vi "figure 8 or loop.vi"() -> ()   [LabVIEW 2014]
doc: "\"Discrete LED demo.vi\" -- Demonstrate a discrete LED connected to a digital output.\n\nInstructions:\n\n-- Click the 'enable blinker' button to toggle between blinking mode\nand static mode.\n-- In static mode, click the 'digital level' button to set the state of the\ndigital output.\n-- The 'digital output state' LED indicator shows the state of the\ndigital output (on = high, off = low)."
uses:
  <vilib>/myRIO/Common/Instrument Driver Framework/myRIO v1.0/UART/vis/myRIO v1.0 Close UART.vi
  <vilib>/Utility/error.llb/Error Cluster From Error Code.vi
  <vilib>/myRIO/Common/Instrument Driver Framework/myRIO v1.0/DIO/vis/myRIO v1.0 Write DIO.vi
  <vilib>/myRIO/Common/Instrument Driver Framework/Utilities/vis/FPGA Ref Manager.vi
  <vilib>/myRIO/Common/Instrument Driver Framework/myRIO v1.0/myRIO v1.0 Reset FPGA.vi
  <vilib>/myRIO/Common/Instrument Driver Framework/myRIO v1.0/IRQ/vis/myRIO v1.0 IRQ Info FGV.vi
  <vilib>/myRIO/Common/Instrument Driver Framework/myRIO v1.0/IRQ/vis/myRIO v1.0 Timer IRQ Info FGV.vi
  <vilib>/myRIO/Common/Instrument Driver Framework/myRIO v1.0/IRQ/vis/myRIO v1.0 ISR Agent.vi
  <vilib>/myRIO/Instrument Drivers/Utilities/Utilities.lvlib
  <vilib>/myRIO/Instrument Drivers/Onboard IO/DIO/DIO.lvlib
panel:
  in  "Numeric":dbl
  in  "reverse":bool
  in  "figure 8":bool
  in  "error in (no error)":errorcluster
  in  "[ESC]":bool
  # "7-Segment LED demo"
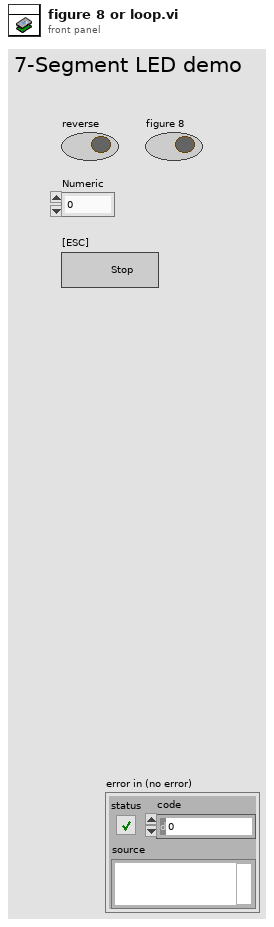
[diagram p1: front panel]
types:
  T1 = typedef "DIO.lvlib/DIO Reference.ctl" = cluster{"myRIO Reference":T2, "DIO Channels List":T6}
  T2 = typedef "myRIO Generic Hardware Reference.ctl" = cluster{"myRIO Model":T3, "myRIO Hardware Reference":T4}
  T3 = typedef "Hardware Version Enum.ctl" = enum16{"Unknown", "myRIO-1900", "myRIO-1950"}
  T4 = typedef "myRIO v1.0 Reference.ctl" = cluster{"Generic FPGA Reference":T5, "Allow multiple opens":bool}
  T5 = typedef "Generic FPGA Reference.ctl" = refnum<k20>
  T6 = typedef "DIO Channels List.ctl" = T7[]
  T7 = typedef "DIO Channels Enum.ctl" = enum16{"Not Connected", "C/DIO0", "C/DIO1", "C/DIO2", "C/DIO3", "C/DIO4", "C/DIO5", "C/DIO6", "C/DIO7", "A/DIO0", "A/DIO1", "A/DIO2", "A/DIO3", "A/DIO4", "A/DIO5", "A/DIO6", "A/DIO7", "A/DIO8", "A/DIO9", "A/DIO10", "A/DIO11", "A/DIO12", "A/DIO13", "A/DIO14", "A/DIO15", "B/DIO0", "B/DIO1", "B/DIO2", "B/DIO3", "B/DIO4", "B/DIO5", "B/DIO6", "B/DIO7", "B/DIO8", "B/DIO9", "B/DIO10", "B/DIO11", "B/DIO12", "B/DIO13", "B/DIO14", "B/DIO15", "LED0", "LED1", "LED2", "LED3", "Button0"}
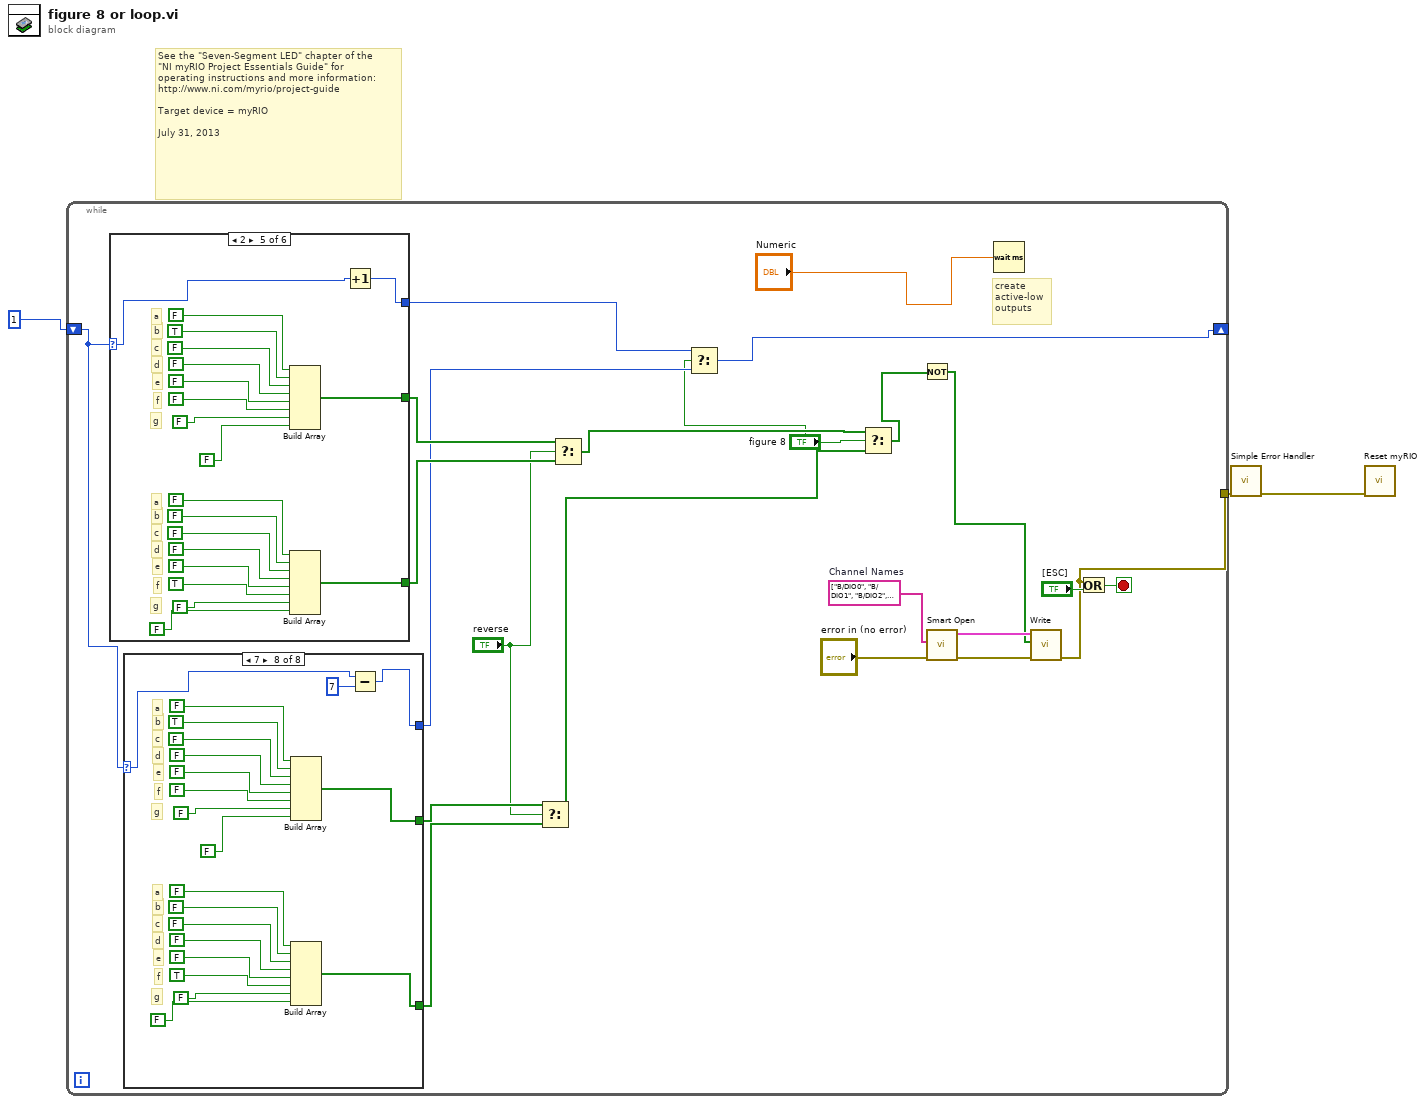
[diagram p0: block diagram]
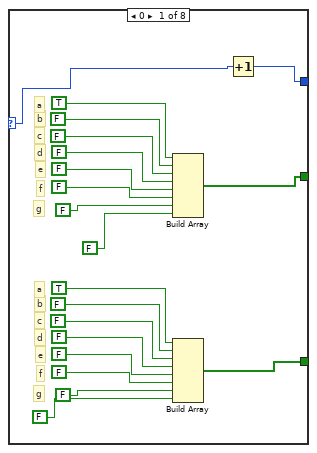
[diagram p2: hidden frame]
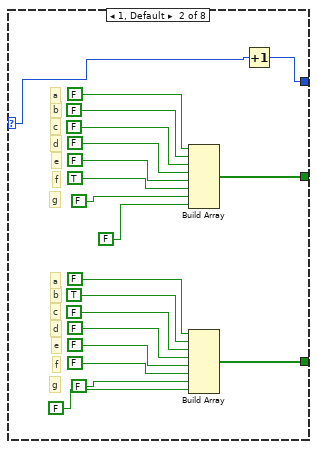
[diagram p3: hidden frame]
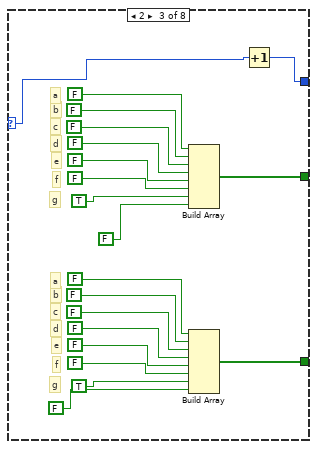
[diagram p4: hidden frame]
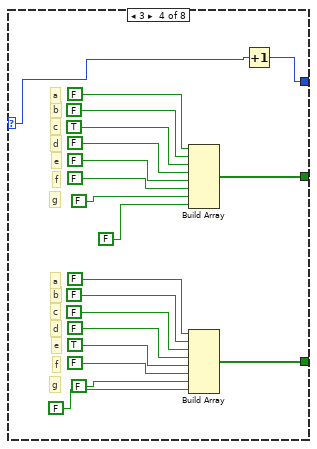
[diagram p5: hidden frame]
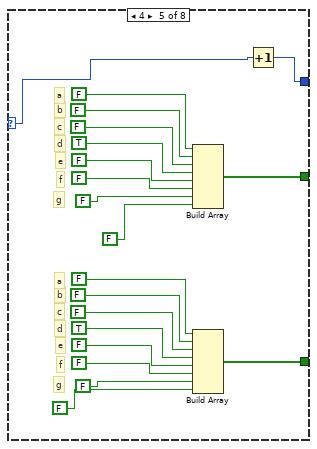
[diagram p6: hidden frame]
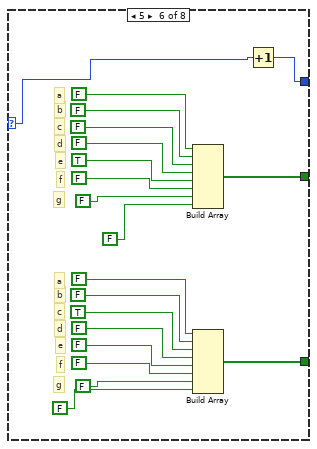
[diagram p7: hidden frame]
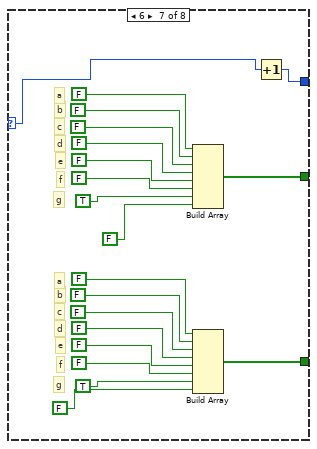
[diagram p8: hidden frame]
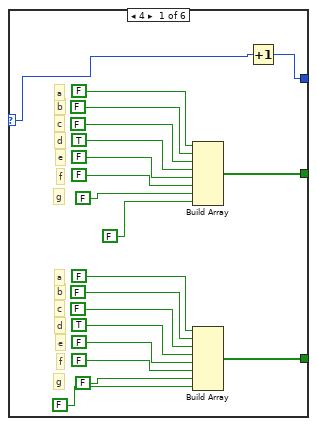
[diagram p9: hidden frame]
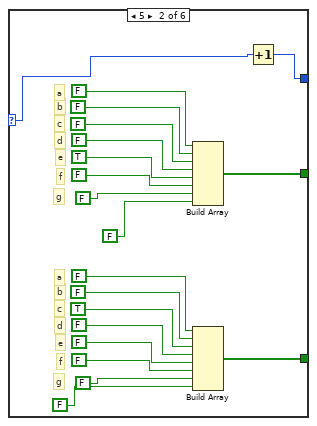
[diagram p10: hidden frame]
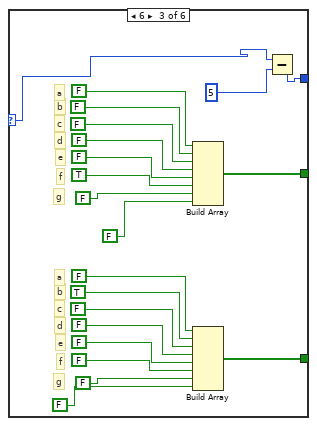
[diagram p11: hidden frame]
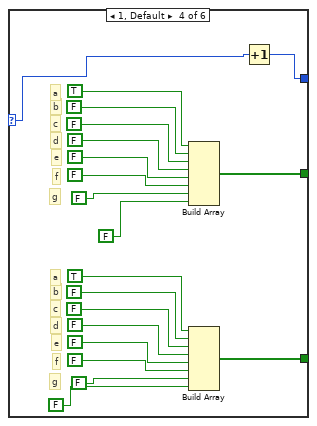
[diagram p12: hidden frame]
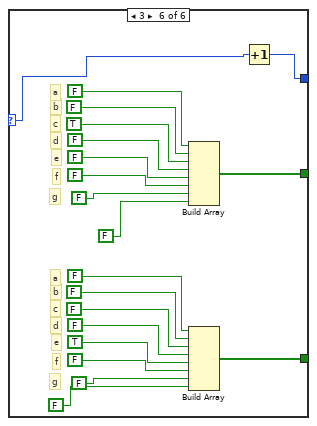
[diagram p13: hidden frame]
diagram:
  # "See the \"Seven-Segment LED\" chapter of the\n\"NI myRIO Project Essentials Guide\" for\noperating instructions and more information: \nhttp://www.ni.com/myrio/project-guide\n\nTarget device = myRIO\n\nJuly 31, 2013"
  n1 = while {
    tunnel: [w19] -> w3
    shift-right: [w7] -> _
    shift-left: 1 -> [w16]
    stop <- w25 stop-if-true
    w23 = tag[] ["B/DIO0", "B/DIO1", "B/DIO2", "B/DIO3", "B/DIO4", "B/DIO5", "B/DIO6", "B/DIO7"]  # Channel Names
    # "create\nactive-low\noutputs"
    n2 = case shown="2" w16 {
      selector: w16 -> [w189 w209 w229 w248 w268 w288]
      tunnel: [w198 w218 w228 w249 w269 w289] -> w8
      tunnel: [w188 w208 w231 w251 w271 w291] -> w11
      tunnel: [w187 w207 w230 w250 w270 w290] -> w10
      frame 4 {
        # "g"
        # "f"
        # "e"
        # "d"
        # "c"
        # "b"
        # "a"
        # "g"
        # "f"
        # "e"
        # "d"
        # "c"
        # "b"
        # "a"
        n3 = Build Array(FALSE, FALSE, FALSE, TRUE, FALSE, FALSE, FALSE, FALSE) -> (w187:bool[])
        n4 = Build Array(FALSE, FALSE, FALSE, TRUE, FALSE, FALSE, FALSE, FALSE) -> (w188:bool[])
        n5 = Increment(x=w189) -> (x+1=w198:i32)
      }
      frame 5 {
        # "g"
        # "f"
        # "e"
        # "d"
        # "c"
        # "b"
        # "a"
        # "g"
        # "f"
        # "e"
        # "d"
        # "c"
        # "b"
        # "a"
        n6 = Build Array(FALSE, FALSE, FALSE, FALSE, TRUE, FALSE, FALSE, FALSE) -> (w207:bool[])
        n7 = Build Array(FALSE, FALSE, TRUE, FALSE, FALSE, FALSE, FALSE, FALSE) -> (w208:bool[])
        n8 = Increment(x=w209) -> (x+1=w218:i32)
      }
      frame 6 {
        # "g"
        # "f"
        # "e"
        # "d"
        # "c"
        # "b"
        # "a"
        # "g"
        # "f"
        # "e"
        # "d"
        # "c"
        # "b"
        # "a"
        n9 = Build Array(FALSE, FALSE, FALSE, FALSE, FALSE, TRUE, FALSE, FALSE) -> (w230:bool[])
        n10 = Build Array(FALSE, TRUE, FALSE, FALSE, FALSE, FALSE, FALSE, FALSE) -> (w231:bool[])
        n11 = Subtract(x=w229, y=5) -> (x-y=w228:i32)
      }
      frame 1, Default {
        # "g"
        # "f"
        # "e"
        # "d"
        # "c"
        # "b"
        # "a"
        # "g"
        # "f"
        # "e"
        # "d"
        # "c"
        # "b"
        # "a"
        n12 = Build Array(TRUE, FALSE, FALSE, FALSE, FALSE, FALSE, FALSE, FALSE) -> (w250:bool[])
        n13 = Build Array(TRUE, FALSE, FALSE, FALSE, FALSE, FALSE, FALSE, FALSE) -> (w251:bool[])
        n14 = Increment(x=w248) -> (x+1=w249:i32)
      }
      frame 2 {
        # "g"
        # "f"
        # "e"
        # "d"
        # "c"
        # "b"
        # "a"
        # "g"
        # "f"
        # "e"
        # "d"
        # "c"
        # "b"
        # "a"
        n15 = Build Array(FALSE, TRUE, FALSE, FALSE, FALSE, FALSE, FALSE, FALSE) -> (w270:bool[])
        n16 = Build Array(FALSE, FALSE, FALSE, FALSE, FALSE, TRUE, FALSE, FALSE) -> (w271:bool[])
        n17 = Increment(x=w268) -> (x+1=w269:i32)
      }
      frame 3 {
        # "g"
        # "f"
        # "e"
        # "d"
        # "c"
        # "b"
        # "a"
        # "g"
        # "f"
        # "e"
        # "d"
        # "c"
        # "b"
        # "a"
        n18 = Build Array(FALSE, FALSE, TRUE, FALSE, FALSE, FALSE, FALSE, FALSE) -> (w290:bool[])
        n19 = Build Array(FALSE, FALSE, FALSE, FALSE, TRUE, FALSE, FALSE, FALSE) -> (w291:bool[])
        n20 = Increment(x=w288) -> (x+1=w289:i32)
      }
    }
    n21 = case shown="7" w16 {
      selector: w16 -> [w26 w46 w66 w86 w108 w128 w147 w168]
      tunnel: [w27 w47 w67 w87 w117 w137 w146 w167] -> w9
      tunnel: [w28 w49 w69 w89 w107 w127 w149 w169] -> w15
      tunnel: [w29 w48 w68 w88 w106 w126 w148 w170] -> w14
      frame 0 {
        # "g"
        # "f"
        # "e"
        # "d"
        # "c"
        # "b"
        # "a"
        # "g"
        # "f"
        # "e"
        # "d"
        # "c"
        # "b"
        # "a"
        n22 = Build Array(TRUE, FALSE, FALSE, FALSE, FALSE, FALSE, FALSE, FALSE) -> (w29:bool[])
        n23 = Build Array(TRUE, FALSE, FALSE, FALSE, FALSE, FALSE, FALSE, FALSE) -> (w28:bool[])
        n24 = Increment(x=w26) -> (x+1=w27:i32)
      }
      frame 1, Default {
        # "g"
        # "f"
        # "e"
        # "d"
        # "c"
        # "b"
        # "a"
        # "g"
        # "f"
        # "e"
        # "d"
        # "c"
        # "b"
        # "a"
        n25 = Build Array(FALSE, FALSE, FALSE, FALSE, FALSE, TRUE, FALSE, FALSE) -> (w48:bool[])
        n26 = Build Array(FALSE, TRUE, FALSE, FALSE, FALSE, FALSE, FALSE, FALSE) -> (w49:bool[])
        n27 = Increment(x=w46) -> (x+1=w47:i32)
      }
      frame 2 {
        # "g"
        # "f"
        # "e"
        # "d"
        # "c"
        # "b"
        # "a"
        # "g"
        # "f"
        # "e"
        # "d"
        # "c"
        # "b"
        # "a"
        n28 = Build Array(FALSE, FALSE, FALSE, FALSE, FALSE, FALSE, TRUE, FALSE) -> (w68:bool[])
        n29 = Build Array(FALSE, FALSE, FALSE, FALSE, FALSE, FALSE, TRUE, FALSE) -> (w69:bool[])
        n30 = Increment(x=w66) -> (x+1=w67:i32)
      }
      frame 3 {
        # "g"
        # "f"
        # "e"
        # "d"
        # "c"
        # "b"
        # "a"
        # "g"
        # "f"
        # "e"
        # "d"
        # "c"
        # "b"
        # "a"
        n31 = Build Array(FALSE, FALSE, TRUE, FALSE, FALSE, FALSE, FALSE, FALSE) -> (w88:bool[])
        n32 = Build Array(FALSE, FALSE, FALSE, FALSE, TRUE, FALSE, FALSE, FALSE) -> (w89:bool[])
        n33 = Increment(x=w86) -> (x+1=w87:i32)
      }
      frame 4 {
        # "g"
        # "f"
        # "e"
        # "d"
        # "c"
        # "b"
        # "a"
        # "g"
        # "f"
        # "e"
        # "d"
        # "c"
        # "b"
        # "a"
        n34 = Build Array(FALSE, FALSE, FALSE, TRUE, FALSE, FALSE, FALSE, FALSE) -> (w106:bool[])
        n35 = Build Array(FALSE, FALSE, FALSE, TRUE, FALSE, FALSE, FALSE, FALSE) -> (w107:bool[])
        n36 = Increment(x=w108) -> (x+1=w117:i32)
      }
      frame 5 {
        # "g"
        # "f"
        # "e"
        # "d"
        # "c"
        # "b"
        # "a"
        # "g"
        # "f"
        # "e"
        # "d"
        # "c"
        # "b"
        # "a"
        n37 = Build Array(FALSE, FALSE, FALSE, FALSE, TRUE, FALSE, FALSE, FALSE) -> (w126:bool[])
        n38 = Build Array(FALSE, FALSE, TRUE, FALSE, FALSE, FALSE, FALSE, FALSE) -> (w127:bool[])
        n39 = Increment(x=w128) -> (x+1=w137:i32)
      }
      frame 6 {
        # "g"
        # "f"
        # "e"
        # "d"
        # "c"
        # "b"
        # "a"
        # "g"
        # "f"
        # "e"
        # "d"
        # "c"
        # "b"
        # "a"
        n40 = Build Array(FALSE, FALSE, FALSE, FALSE, FALSE, FALSE, TRUE, FALSE) -> (w148:bool[])
        n41 = Build Array(FALSE, FALSE, FALSE, FALSE, FALSE, FALSE, TRUE, FALSE) -> (w149:bool[])
        n42 = Increment(x=w147) -> (x+1=w146:i32)
      }
      frame 7 {
        # "g"
        # "f"
        # "e"
        # "d"
        # "c"
        # "b"
        # "a"
        # "g"
        # "f"
        # "e"
        # "d"
        # "c"
        # "b"
        # "a"
        n43 = Build Array(FALSE, TRUE, FALSE, FALSE, FALSE, FALSE, FALSE, FALSE) -> (w170:bool[])
        n44 = Build Array(FALSE, FALSE, FALSE, FALSE, FALSE, TRUE, FALSE, FALSE) -> (w169:bool[])
        n45 = Subtract(x=w168, y=7) -> (x-y=w167:i32)
      }
    }
    n46 = Select(t=w14, s="reverse", f=w15) -> (s? t:f=w13:bool[])
    n47 = Select(t=w10, s="reverse", f=w11) -> (s? t:f=w12:bool[])
    n48 = Select(t=w8, s="figure 8", f=w9) -> (s? t:f=w7:i32)
    n49 = Select(t=w12, s="figure 8", f=w13) -> (s? t:f=w17:bool[])
    n50 = Not(x=w17) -> (.not. x?=w18:bool[])
    n51 = call <vilib>:"Smart Open.vi"("error in (no error)"="error in (no error)", "Channel Names"=w23) -> ("error out"=w20:errorcluster, "DIO Ref Out"=w21:T1)  [unwired: 8 in]
    n52 = Wait (ms)(milliseconds to wait="Numeric") -> ()  [unwired: 1 out]
    n53 = call <vilib>:"Write.vi"("error in (no error)"=w20, "Values"=w18, "DIO Ref In"=w21) -> ("error out"=w19:errorcluster)  [unwired: 6 in, 1 out]
    n54 = Or(x=w19, y="[ESC]") -> (x .or. y?=w25:bool)
  }
  n55 = call <vilib>:"Simple Error Handler.vi"("error in (no error)"=w3) -> ("error out"=w2:errorcluster)  [unwired: 4 in, 4 out]
  n56 = call <vilib>:"Reset myRIO.vi"("error in (no error)"=w2) -> ()  [unwired: 10 in, 1 out]
